vi "Get PID Controllers.vi"(8 "error in (no error)":errorcluster, 11 "Item Ref in":T1 format="%.0x") -> (0 "error out":errorcluster, 2 "PID Settings":T2 {"Read Refs"."Data Reference" format="%.0x"; "Write Refs"."Data Reference" format="%.0x"}, 3 "Device Ref out":T1 format="%.0x")   [LabVIEW 2019, in "Control Addon System Explorer.lvlib"]
uses:
  Control Addon System Explorer.lvlib
  <vilib>/NI VeriStand/Custom Device API/Custom Device Item Ref.ctl
  Addon Shared/Types/Compiled PID Settings.ctl
  Addon Shared/Types/Gain Schedule.ctl
  <vilib>/NI VeriStand/Custom Device API/Block Data Reference.ctl
  <vilib>/NI VeriStand/Custom Device API/Data Reference.ctl
  <vilib>/NI VeriStand/Custom Device API/Data Access Type.ctl
  Types/Action.ctl
  Addon Shared/SubVIs/Constants.vi
  <vilib>/NI VeriStand/Custom Device Tools/Custom Device Utility Library/NI VeriStand - Search for All Items by GUID.vi
  <vilib>/NI VeriStand/Custom Device API/Get Item Property (Double).vi
  <vilib>/NI VeriStand/Custom Device API/Get Item Property (Boolean).vi
  <vilib>/NI VeriStand/Custom Device API/NI VeriStand - Set Item Property.vi
  <vilib>/NI VeriStand/Custom Device API/Set Item Property (Double).vi
  <vilib>/NI VeriStand/Custom Device API/Set Item Property (Boolean).vi
  <vilib>/NI VeriStand/Custom Device API/Get Item Property (Dependent Node Pointer).vi
  <vilib>/NI VeriStand/Custom Device Tools/Custom Device Utility Library/NI VeriStand - Search for Item by GUID.vi
  <vilib>/NI VeriStand/Custom Device API/Get Item Property (String).vi
  <vilib>/NI VeriStand/Custom Device API/Set Item Property (String).vi
  Addon Shared/Control Addon Shared.lvlib
  <vilib>/NI VeriStand/Custom Device API/Custom Device API.lvlib
  <vilib>/NI VeriStand/Custom Device Tools/Custom Device Utility Library/Custom Device Utility Library.lvlib
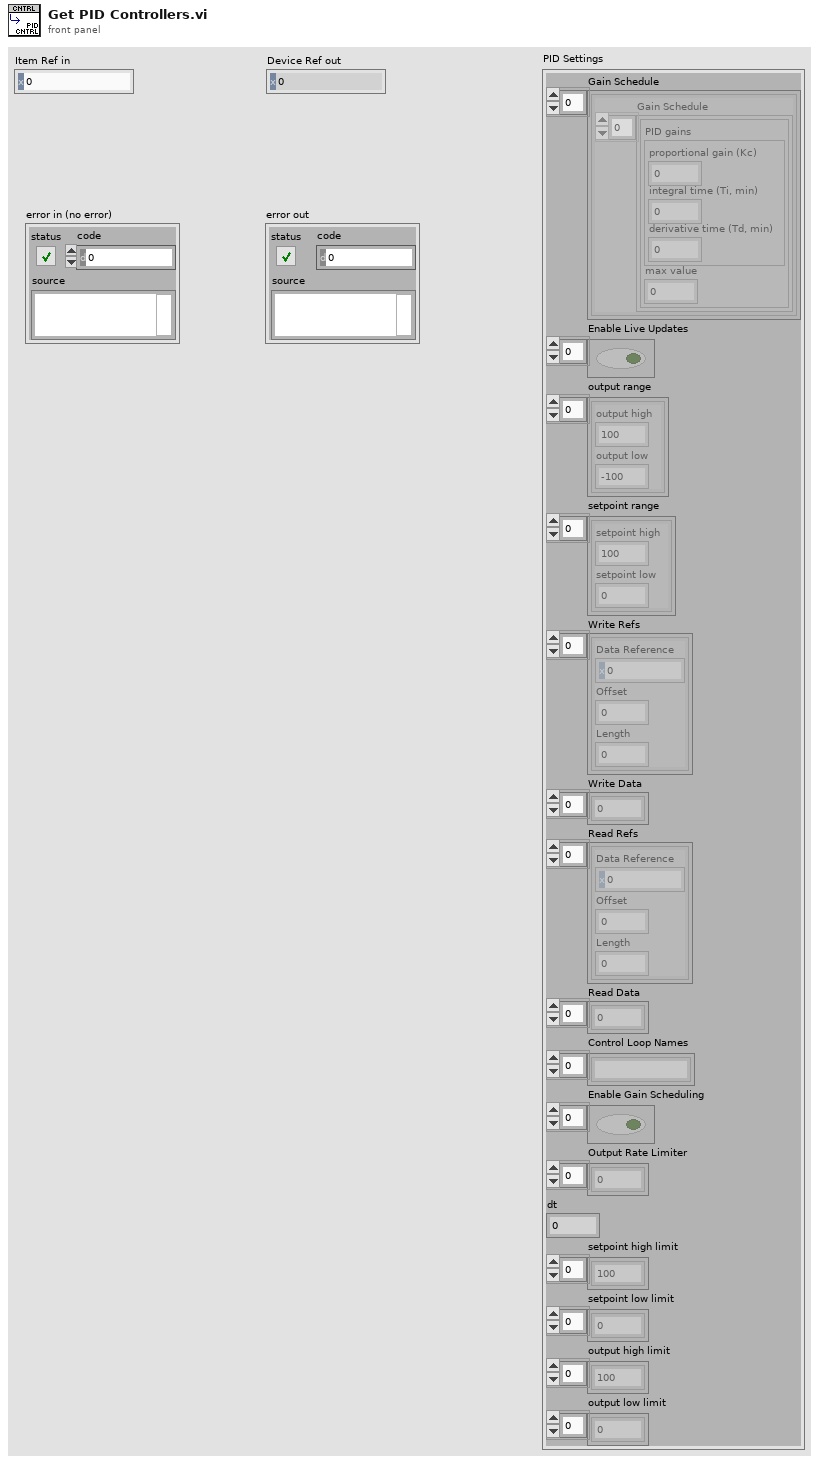
[diagram p1: front panel]
types:
  T1 = typedef "Custom Device API.lvlib/Custom Device Item Ref.ctl" = u64
  T2 = typedef "Control Addon Shared.lvlib/Compiled PID Settings.ctl" = cluster{"Gain Schedule":T3[], "Enable Live Updates":bool[], "output range":cluster{"output high":dbl, "output low":dbl}[], "setpoint range":cluster{"setpoint high":dbl, "setpoint low":dbl}[], "Write Refs":T4[], "Write Data":dbl[], "Read Refs":T4[], "Read Data":dbl[], "Control Loop Names":string[], "Enable Gain Scheduling":bool[], "Output Rate Limiter":dbl[], "dt":dbl, "setpoint high limit":dbl[], "setpoint low limit":dbl[], "output high limit":dbl[], "output low limit":dbl[]}
  T3 = typedef "Control Addon Shared.lvlib/Gain Schedule.ctl" = cluster{"Gain Schedule":cluster{"PID gains":cluster{"proportional gain (Kc)":dbl, "integral time (Ti, min)":dbl, "derivative time (Td, min)":dbl}, "max value":dbl}[]}
  T4 = typedef "Custom Device API.lvlib/Block Data Reference.ctl" = cluster{"Data Reference":T5, "Offset":u64, "Length":u64}
  T5 = typedef "Custom Device API.lvlib/Data Reference.ctl" = i32
  T6 = typedef "Custom Device API.lvlib/Data Access Type.ctl" = enum16{"Read", "Write"}
  T7 = typedef "Control Addon System Explorer.lvlib/Action.ctl" = enum16{"Get", "Set"}
  T8 = cluster{"PID gains":cluster{"proportional gain (Kc)":dbl, "integral time (Ti, min)":dbl, "derivative time (Td, min)":dbl}, "max value":dbl}
  T9 = typedef "Custom Device API.lvlib/Custom Device Item Info.ctl" = cluster{"Name":string, "Is Channel":bool, "GUID":string, "Is Waveform":bool}
  T10 = typedef "Control Addon Shared.lvlib/Controller Settings.ctl" = cluster{"Output Max":dbl, "Output Min":dbl, "Setpoint Max":dbl, "Setpoint Min":dbl, "Use External Setpoint":bool, "Output Rate Limiter":dbl}
  T11 = typedef "Control Addon Shared.lvlib/PID Parameters.ctl" = cluster{"Enable Live Updates":bool, "Enable Gain Scheduling":bool, "PID Parameters":dbl[][]}
  T12 = cluster{"PID gains":cluster{"proportional gain (Kc)":dbl, "integral time (Ti, min)":dbl, "derivative time (Td, min)":dbl}, "max value":dbl}[]
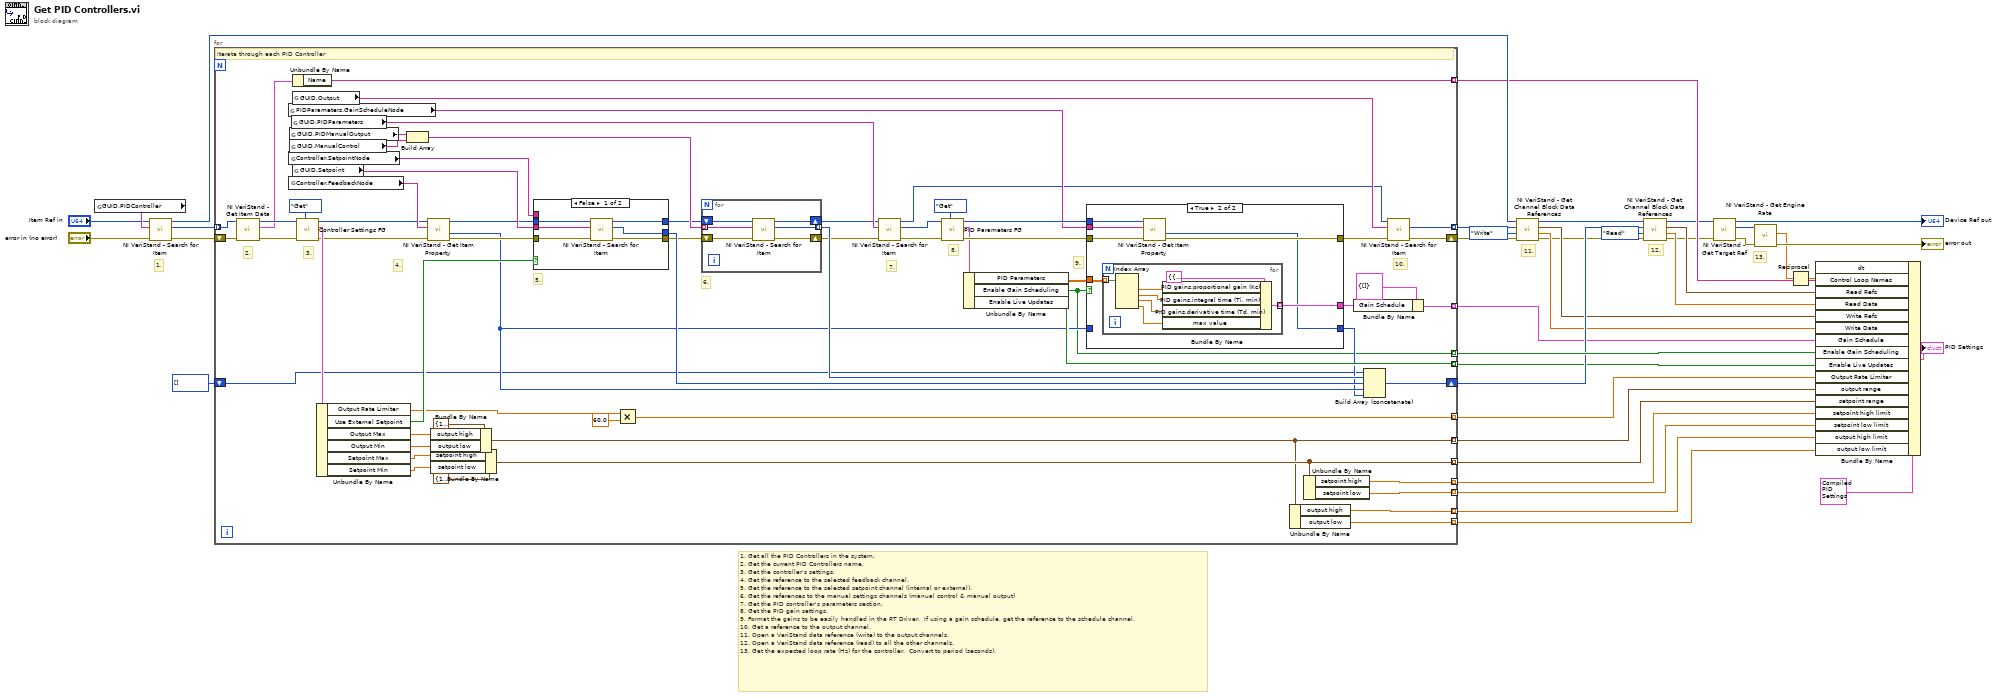
[diagram p0: block diagram]
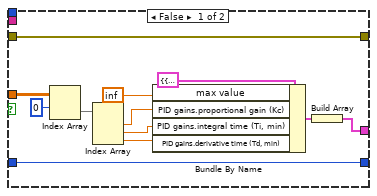
[diagram p2: hidden frame]
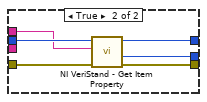
[diagram p3: hidden frame]
diagram:
  # "1. Get all the PID Controllers in the system.\n2. Get the current PID Controllers name.\n3. Get the controller's settings.\n4. Get the reference to the selected feedback channel.\n5. Get the reference to the selected setpoint channel (internal or external).\n6. Get the references to the manual settings channels (manual control & manual output)\n7. Get the PID controller's parameters section.\n8. Get the PID gain settings.\n9. Format the gains to be easily handled in the RT Driver.  If using a gain schedule, get the reference to the schedule channel.\n10. Get a reference to the output channel.\n11. Open a VeriStand data reference (write) to the output channels.\n12. Open a VeriStand data reference (read) to all the other channels. \n13. Get the expected loop rate (Hz) for the controller.  Convert to period (seconds)."
  # "13."
  # "12."
  # "11."
  # "1."
  n1 = global read "Constants.vi" "GUID.PIDController"() -> (w38:string)
  n2 = call-poly <vilib>:"NI VeriStand - Search for Item.vi"("error in"="error in (no error)", "Item GUID"=w38, "Section Ref in"="Item Ref in") -> ("error out"=w35:errorcluster, "Item Refs"=w37:T1[], "Section Ref out"=w36:T1)  [unwired: 5 in, 1 out]
  n3 = for {
    shift-right: [w67] -> w14
    shift-left: w35 -> [w53]
    tunnel: w37 -> [w55] mode=indexing
    tunnel: [w45] -> w27 mode=indexing
    tunnel: [w42] -> w26 mode=indexing
    tunnel: [w65] -> w21 mode=indexing
    tunnel: [w64] -> w16 mode=indexing
    tunnel: [w59] -> w20 mode=indexing
    shift-right: [w62] -> w29
    shift-left: T1[] [] -> [w56]
    tunnel: [w50] -> w31 mode=indexing
    tunnel: [w49] -> w32 mode=indexing
    tunnel: [w47] -> w13 mode=indexing
    tunnel: [w44] -> w4 mode=indexing
    tunnel: [w43] -> w3 mode=indexing
    tunnel: [w41] -> w2 mode=indexing
    tunnel: [w40] -> w1 mode=indexing
    # "10."
    # "9."
    # "8."
    # "7."
    # "6."
    # "5."
    # "4."
    # "3."
    # "2."
    # "Iterate through each PID Controller"
    n4 = call <vilib>:"NI VeriStand - Get Item Data.vi"("error in (no error)"=w53, "Item Ref in"=w55) -> ("error out"=w52:errorcluster, "Item Info"=w51:T9, "Item Ref out"=w54:T1)  [unwired: 6 in, 1 out]
    n5 = global read "Constants.vi" "PIDParameters.GainScheduleNode"() -> (w89:string)
    n6 = global read "Constants.vi" "Controller.SetpointNode"() -> (w100:string)
    n7 = global read "Constants.vi" "Controller.FeedbackNode"() -> (w99:string)
    n8 = global read "Constants.vi" "GUID.PIDManualOutput"() -> (w96:string)
    n9 = global read "Constants.vi" "GUID.ManualControl"() -> (w88:string)
    n10 = global read "Constants.vi" "GUID.PIDParameters"() -> (w93:string)
    n11 = Unbundle By Name(w51) -> ("Name"=w50:string)
    n12 = global read "Constants.vi" "GUID.Output"() -> (w86:string)
    n13 = global read "Constants.vi" "GUID.Setpoint"() -> (w98:string)
    n14 = call "Controller Settings FG.vi"("Action"=Action."Get", "error in (no error)"=w52, "Node Ptr"=w54) -> ("error out"=w73:errorcluster, "Controller Settings"=w81:T10, "Item Ref out"=w72:T1)  [unwired: 6 in]
    n15 = Unbundle By Name(w81) -> ("Output Rate Limiter"=w48:dbl, "Use External Setpoint"=w101:bool, "Output Max"=w75:dbl, "Output Min"=w76:dbl, "Setpoint Max"=w77:dbl, "Setpoint Min"=w78:dbl)
    n16 = Build Array(w96, w88) -> (w97:string[])
    n17 = call-poly <vilib>:"NI VeriStand - Get Item Property.vi"("error in (no error)"=w73, "Property Name"=w99, "Item Ref in"=w72) -> ("error out"=w70:errorcluster, "Dependent Node Ref"=w58:T1, "Item Ref out"=w71:T1)  [unwired: 5 in, 1 out]
    n18 = Bundle By Name(cluster=cluster{"output high":dbl, "output low":dbl} {"output high"=100.0, "output low"=-100.0} ("output range"), "output high"=w75, "output low"=w76) -> (w42:cluster{"output high":dbl, "output low":dbl})
    n19 = Bundle By Name(cluster=cluster{"setpoint high":dbl, "setpoint low":dbl} {"setpoint high"=100.0, "setpoint low"=0.0} ("setpoint range"), "setpoint high"=w77, "setpoint low"=w78) -> (w45:cluster{"setpoint high":dbl, "setpoint low":dbl})
    n20 = case shown="False" w101 {
      tunnel: w70 -> [w140 w146]
      tunnel: w71 -> [w137 w145]
      tunnel: [w139 w144] -> w69
      tunnel: [w138 w143] -> w68
      tunnel: w100 -> [_ w142]
      tunnel: [w135 w141] -> w74
      tunnel: w98 -> [w136 _]
      frame False {
        n21 = call-poly <vilib>:"NI VeriStand - Search for Item.vi"("error in"=w140, "Item GUID"=w136, "Section Ref in"=w137) -> ("error out"=w139:errorcluster, "Item Ref"=w135:T1, "Section Ref out"=w138:T1)  [unwired: 5 in, 1 out]
      }
      frame True {
        n22 = call-poly <vilib>:"NI VeriStand - Get Item Property.vi"("error in (no error)"=w146, "Property Name"=w142, "Item Ref in"=w145) -> ("error out"=w144:errorcluster, "Dependent Node Ref"=w141:T1, "Item Ref out"=w143:T1)  [unwired: 5 in, 1 out]
      }
    }
    n23 = Multiply(x=w48, y=60.0) -> (x*y=w47:dbl)
    n24 = for {
      shift-right: [w130] -> w85
      shift-left: w69 -> [w134]
      shift-right: [w132] -> w84
      shift-left: w68 -> [w133]
      tunnel: w97 -> [w131] mode=indexing
      tunnel: [w129] -> w87 mode=indexing
      n25 = call-poly <vilib>:"NI VeriStand - Search for Item.vi"("error in"=w134, "Item GUID"=w131, "Section Ref in"=w133) -> ("error out"=w130:errorcluster, "Item Ref"=w129:T1, "Section Ref out"=w132:T1)  [unwired: 5 in, 1 out]
    }
    n26 = call-poly <vilib>:"NI VeriStand - Search for Item.vi"("error in"=w85, "Item GUID"=w93, "Section Ref in"=w84) -> ("error out"=w95:errorcluster, "Item Ref"=w94:T1, "Section Ref out"=w82:T1)  [unwired: 5 in, 1 out]
    n27 = call "PID Parameters FG.vi"("Action"=Action."Get", "error in (no error)"=w95, "Node Ptr"=w94) -> ("error out"=w91:errorcluster, "Parameters"=w66:T11, "Item Ref out"=w90:T1)  [unwired: 6 in]
    n28 = Unbundle By Name(w66) -> ("PID Parameters"=w63:dbl[][], "Enable Gain Scheduling"=w49:bool, "Enable Live Updates"=w65:bool)
    n29 = case shown="True" w49 {
      tunnel: w91 -> [w114 w121]
      tunnel: [w114 w120] -> w83
      tunnel: w90 -> [_ w119]
      tunnel: w89 -> [_ w118]
      tunnel: [w105 w117] -> w60
      tunnel: w63 -> [w104 w116]
      tunnel: [w103 w115] -> w57
      tunnel: w58 -> [w103 _]
      frame False {
        n30 = Index Array(array=w104, index (row)=0) -> (element=w112:dbl[])  [unwired: 1 in]
        n31 = Index Array(array=w112) -> (element #1=w111:dbl, element #2=w109:dbl, element #3=w110:dbl)  [unwired: 3 in]
        n32 = Bundle By Name(cluster=T8 {"PID gains"={"proportional gain (Kc)"=1.0, "integral time (Ti, min)"=0.01, "derivative time (Td, min)"=0.0}, "max value"=100.0} ("gain schedule"), "max value"=inf, "PID gains.proportional gain (Kc)"=w111, "PID gains.integral time (Ti, min)"=w109, "PID gains.derivative time (Td, min)"=w110) -> (w106:T8)
        n33 = Build Array(w106) -> (w105:T12)
      }
      frame True {
        n34 = for {
          tunnel: w116 -> [w128] mode=indexing
          tunnel: [w122] -> w117 mode=indexing
          n35 = Index Array(array=w128) -> (element #1=w123:dbl, element #2=w124:dbl, element #3=w125:dbl, element #4=w126:dbl)  [unwired: 4 in]
          n36 = Bundle By Name(cluster=T8 {"PID gains"={"proportional gain (Kc)"=1.0, "integral time (Ti, min)"=0.01, "derivative time (Td, min)"=0.0}, "max value"=100.0} ("gain schedule"), "PID gains.proportional gain (Kc)"=w123, "PID gains.integral time (Ti, min)"=w124, "PID gains.derivative time (Td, min)"=w125, "max value"=w126) -> (w122:T8)
        }
        n37 = call-poly <vilib>:"NI VeriStand - Get Item Property.vi"("error in (no error)"=w121, "Property Name"=w118, "Item Ref in"=w119) -> ("error out"=w120:errorcluster, "Dependent Node Ref"=w115:T1)  [unwired: 5 in, 2 out]
      }
    }
    n38 = Unbundle By Name(w42) -> ("output high"=w41:dbl, "output low"=w40:dbl)
    n39 = Unbundle By Name(w45) -> ("setpoint high"=w44:dbl, "setpoint low"=w43:dbl)
    n40 = Bundle By Name(cluster=T3 {"Gain Schedule"=[]}, "Gain Schedule"=w60) -> (w59:T3)
    n41 = Build Array (concatenate)(w56, w87, w74, w58, w57) -> (w62:T1[])
    n42 = call-poly <vilib>:"NI VeriStand - Search for Item.vi"("error in"=w83, "Item GUID"=w86, "Section Ref in"=w82) -> ("error out"=w67:errorcluster, "Item Ref"=w64:T1)  [unwired: 5 in, 2 out]
  }
  n43 = call <vilib>:"NI VeriStand - Get Channel Block Data References.vi"("error in (no error)"=w14, "Access"=Data_Access_Type."Write", "Channel Refs"=w16, "Device Ref in"=w36) -> ("error out"=w15:errorcluster, "Values Array"=w25:dbl[], "Block Data Refs"=w24:T4[], "Device Ref out"=w17:T1)  [unwired: 4 in]
  n44 = call <vilib>:"NI VeriStand - Get Channel Block Data References.vi"("error in (no error)"=w15, "Access"=Data_Access_Type."Read", "Channel Refs"=w29, "Device Ref in"=w17) -> ("error out"=w10:errorcluster, "Values Array"=w23:dbl[], "Block Data Refs"=w22:T4[], "Device Ref out"=w8:T1)  [unwired: 4 in]
  n45 = call <vilib>:"NI VeriStand - Get Target Ref.vi"("error in"=w10, "Item Ref in"=w8) -> ("error out"=w11:errorcluster, "Target Ref"=w12:T1, "Item Ref out"=→"Device Ref out":T1)  [unwired: 6 in, 1 out]
  n46 = call <vilib>:"NI VeriStand - Get Engine Rate.vi"("error in (no error)"=w11, "Item Ref in"=w12) -> ("error out"=→"error out":errorcluster, "Rate (Hz)"=w6:dbl)  [unwired: 7 in, 1 out]
  n47 = Reciprocal(x=w6) -> (1/x=w5:dbl)
  n48 = Bundle By Name(cluster=T2 {"Gain Schedule"=[], "Enable Live Updates"=[], "output range"=[], "setpoint range"=[], "Write Refs"=[], "Write Data"=[], "Read Refs"=[], "Read Data"=[], "Control Loop Names"=[], "Enable Gain Scheduling"=[], "Output Rate Limiter"=[], "dt"=0.0, "setpoint high limit"=[], "setpoint low limit"=[], "output high limit"=[], "output low limit"=[]} ("PID Settings"), "dt"=w5, "Control Loop Names"=w31, "Read Refs"=w22, "Read Data"=w23, "Write Refs"=w24, "Write Data"=w25, "Gain Schedule"=w20, "Enable Gain Scheduling"=w32, "Enable Live Updates"=w21, "Output Rate Limiter"=w13, "output range"=w26, "setpoint range"=w27, "setpoint high limit"=w4, "setpoint low limit"=w3, "output high limit"=w2, "output low limit"=w1) -> (→"PID Settings":T2)
